vi "MPDSnC Engine.vi"(0 "Notifier Name":string, 11 "COM Port":string[](array[string])) -> ()   [LabVIEW 2025]
uses:
  AOTF Controls/AOTF Lines Lines Control.ctl
  AOTF Controls/AOTF Notifier Element.ctl
  AOTF Controls/AOTF Actions.ctl
  <vilib>/Utility/error.llb/Trim Whitespace One-Sided.vi
  <vilib>/Instr/_visa.llb/VISA Configure Serial Port (Instr).vi
panel:
  in  "Line On/Off":bool
  in  "Laser Wavelength (nm)":string
  out "Write Response":string
  in  "Blank":bool
  in  "Quit":bool
  in  "Power":dbl(slide) scale=0.0..100.0
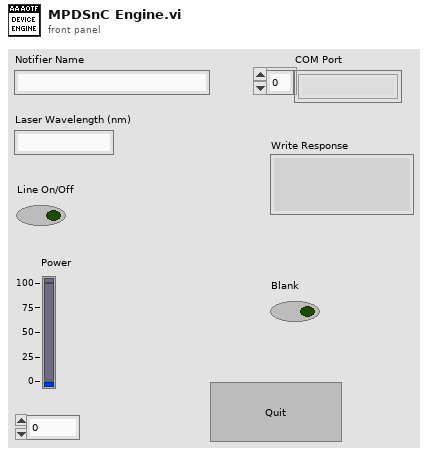
[diagram p1: front panel]
types:
  T1 = typedef "AOTF Notifier Element.ctl" = cluster{"AOTF Action":T2, "Laser Line":string, "Power (%)":dbl, "Beam Blank On/Off":bool, "Line On/Off":bool, "Error":errorcluster, "Wavelengths (nm)":string[]}
  T2 = typedef "AOTF Actions.ctl" = enum16{"Error Check", "Blank", "Line On/Off", "Set Power", "Status", "Quit"}
  T3 = typedef "AOTF Lines Lines Control.ctl" = cluster{"Wavelength":u16[], "AO Line":string[]}
  T4 = enum32{"Invalid", "Standard", "Closed", "Hidden", "Minimized", "Maximized"}
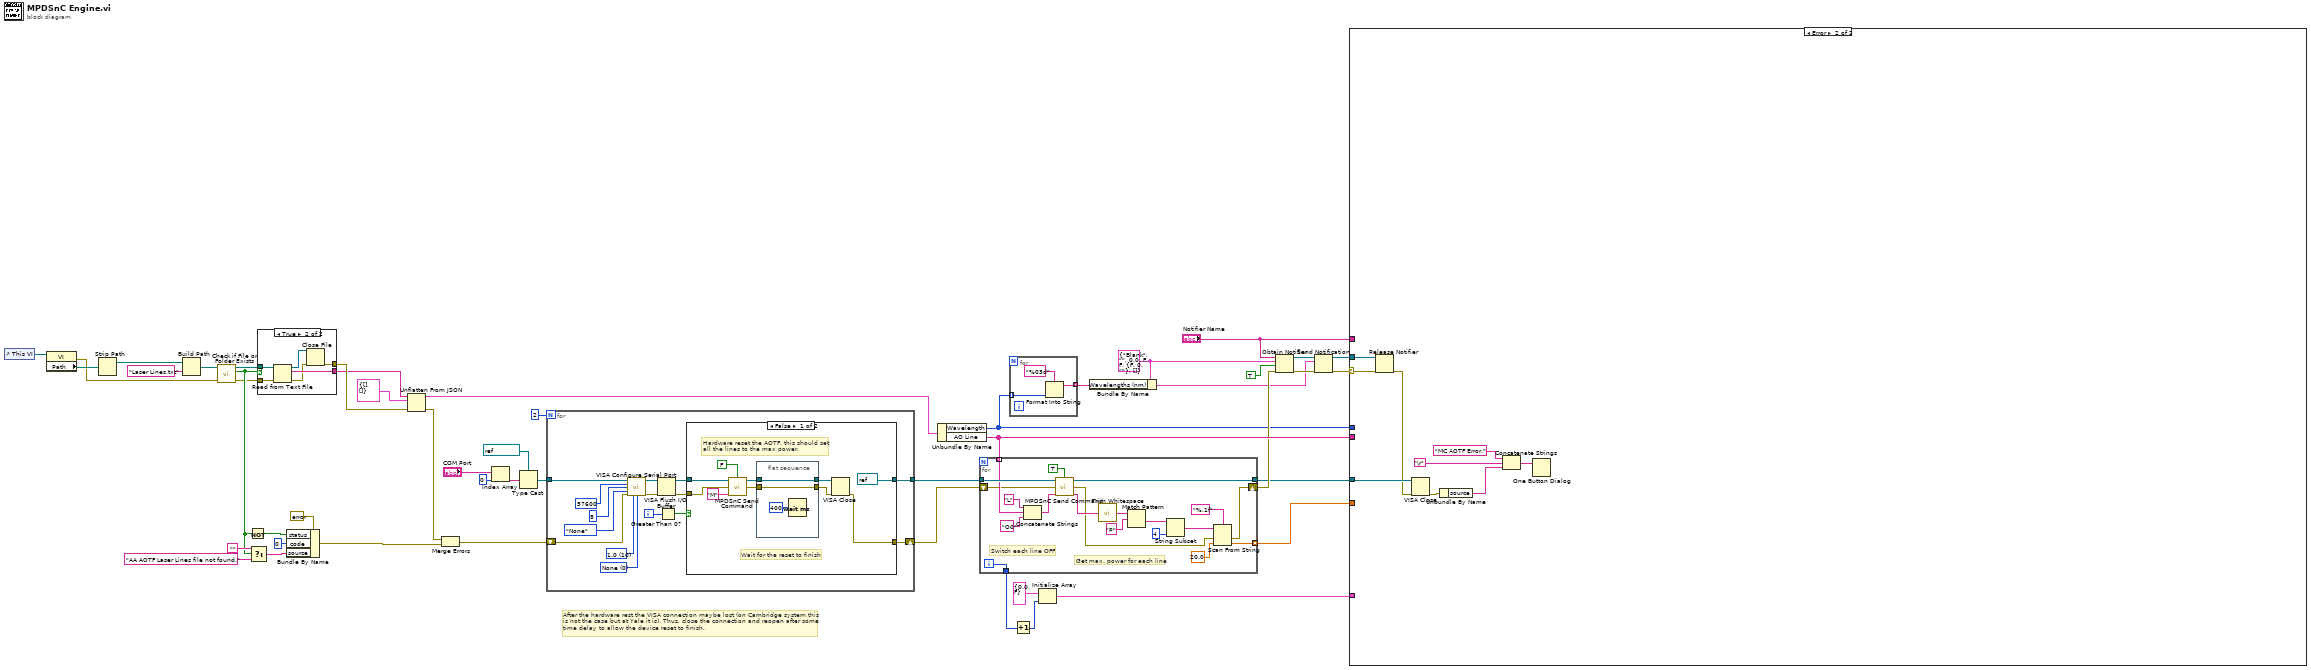
[diagram p0: block diagram]
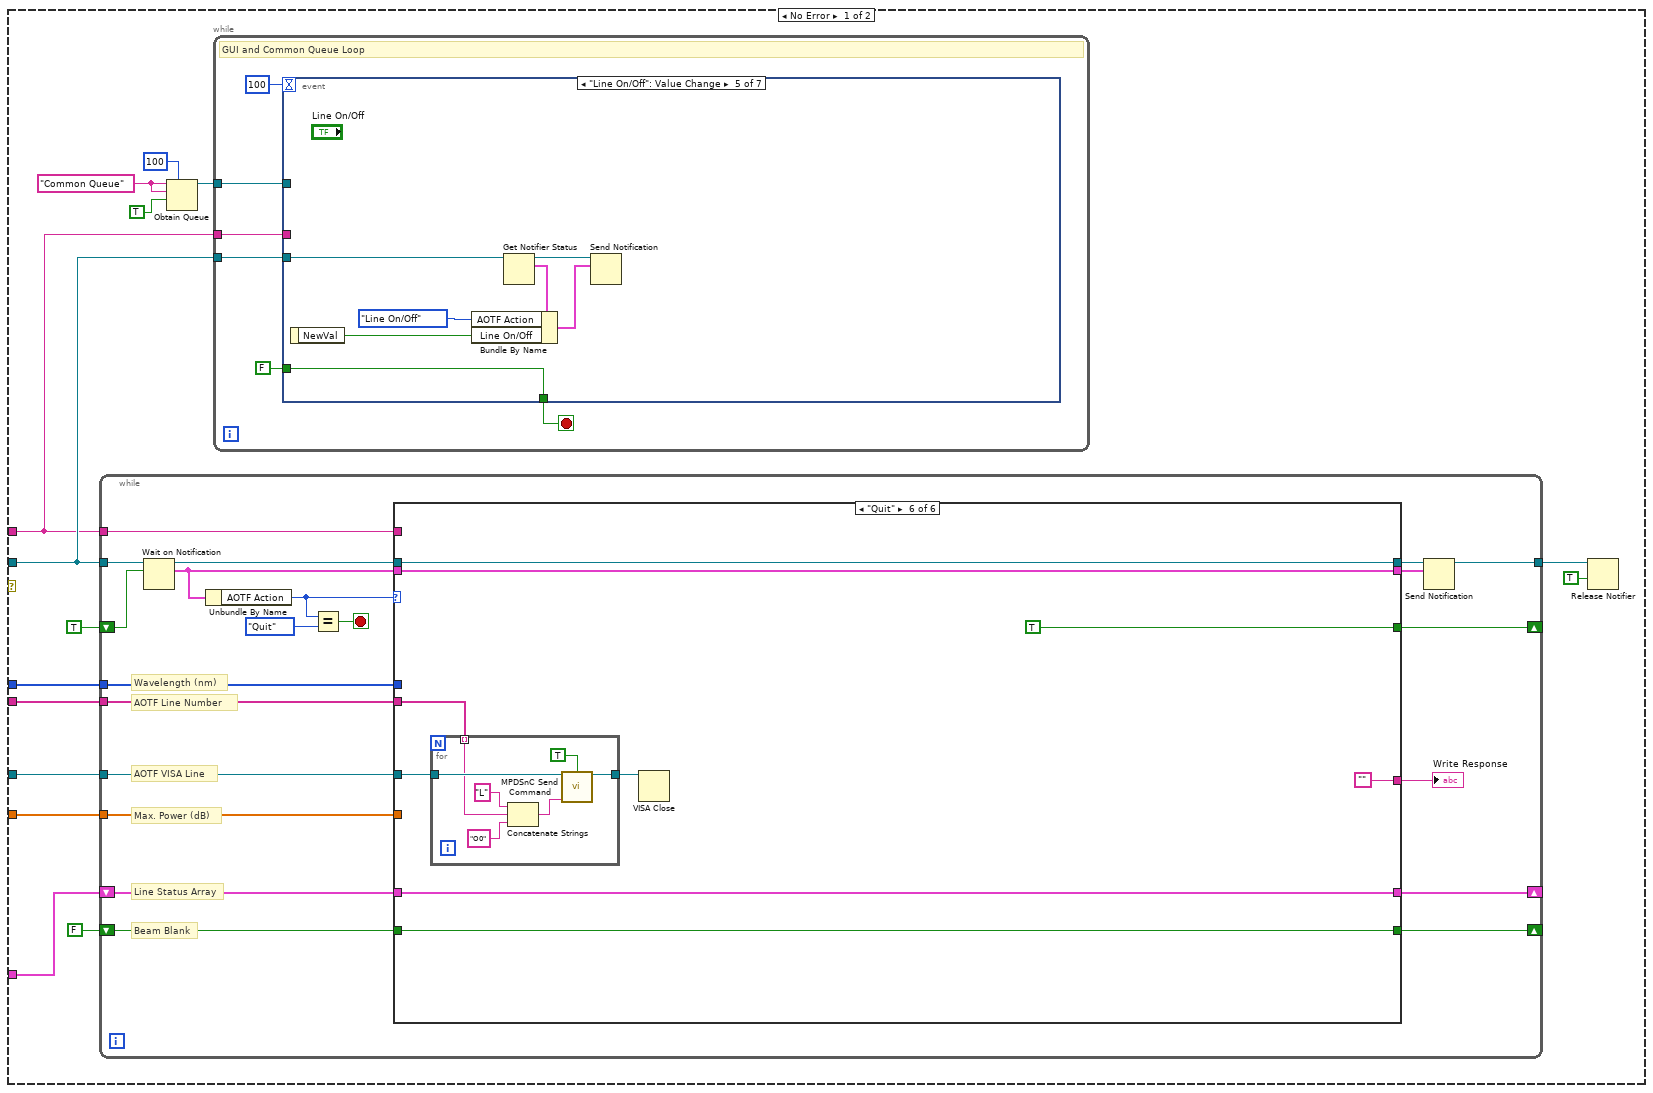
[diagram p3: hidden frame]
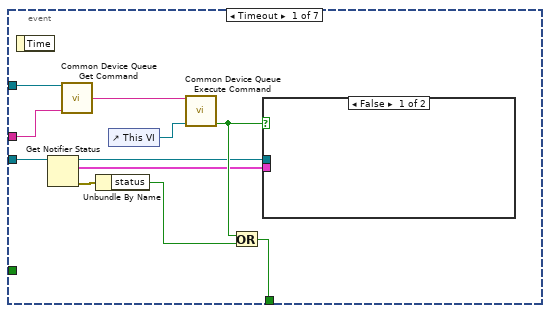
[diagram p4: hidden frame]
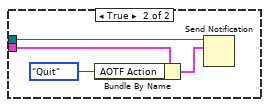
[diagram p5: hidden frame]
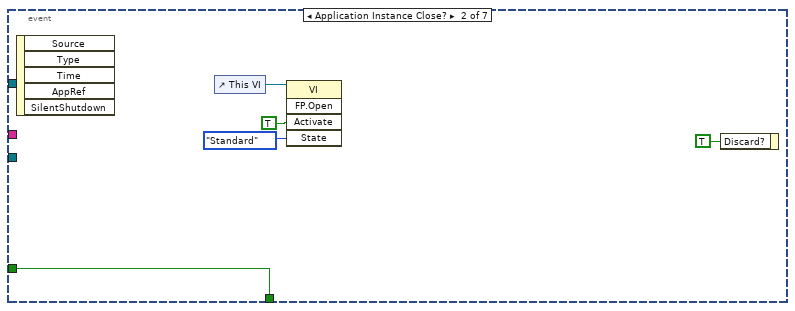
[diagram p6: hidden frame]
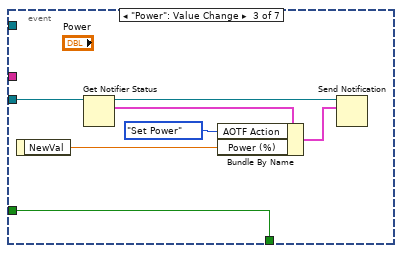
[diagram p7: hidden frame]
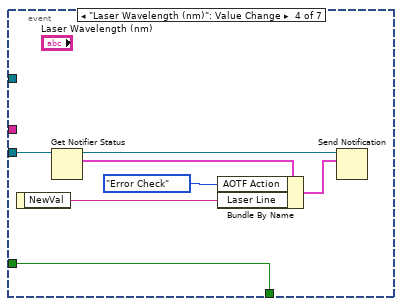
[diagram p8: hidden frame]
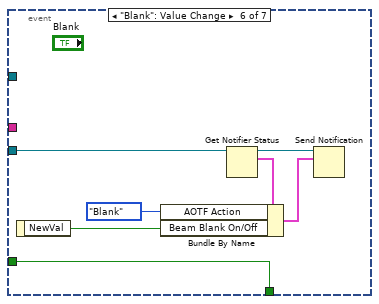
[diagram p9: hidden frame]
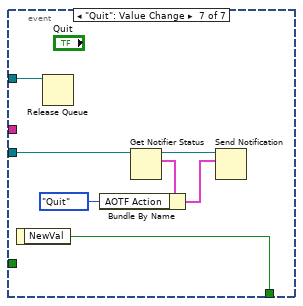
[diagram p10: hidden frame]
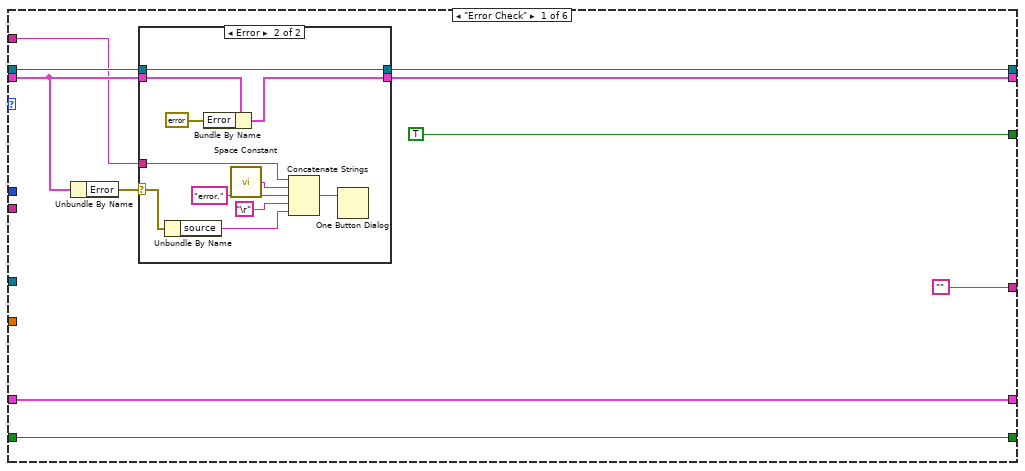
[diagram p11: hidden frame]
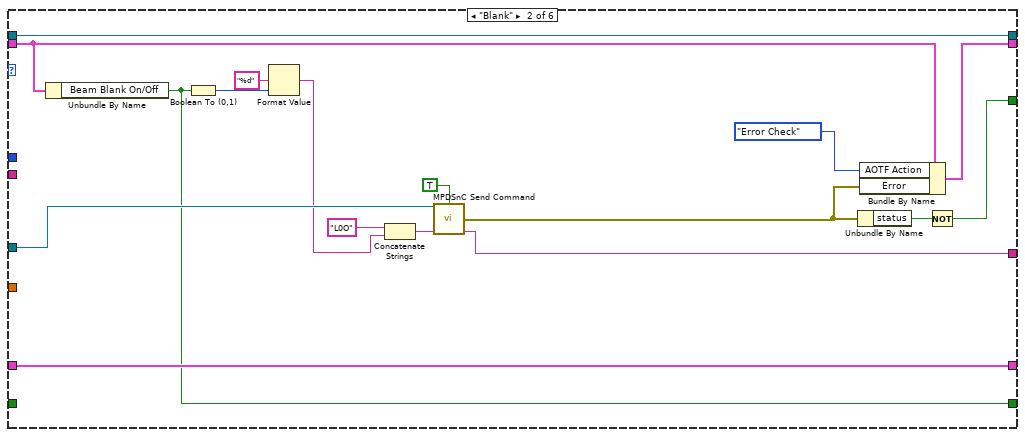
[diagram p13: hidden frame]
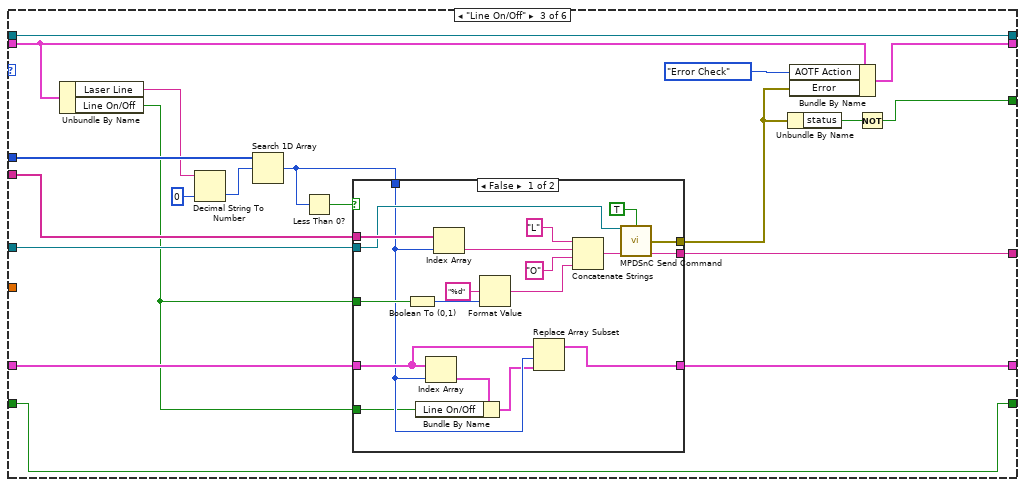
[diagram p14: hidden frame]
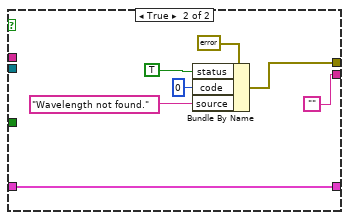
[diagram p15: hidden frame]
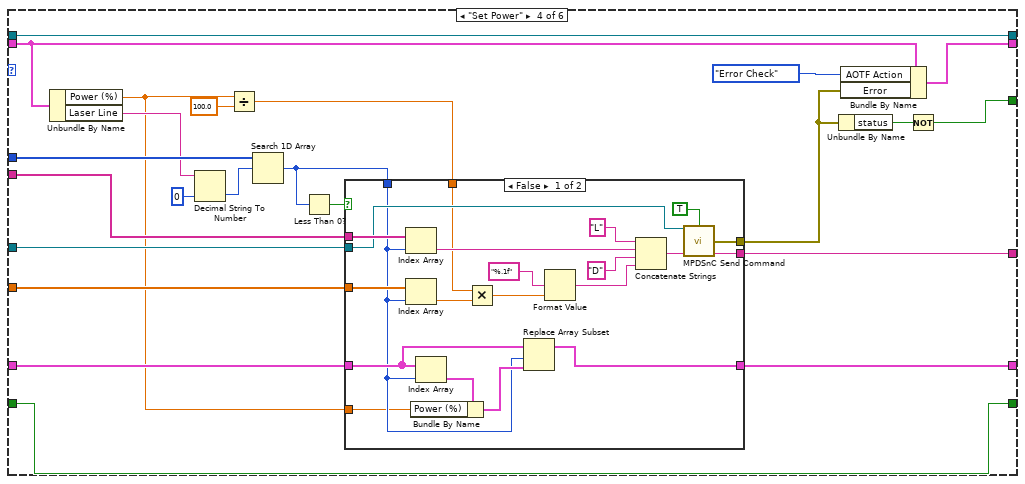
[diagram p16: hidden frame]
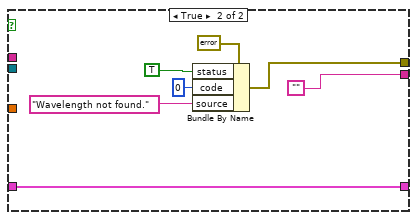
[diagram p17: hidden frame]
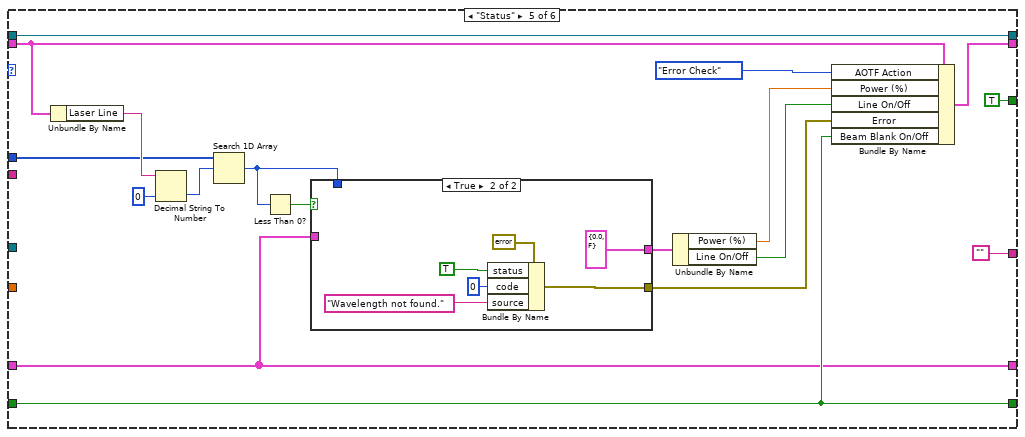
[diagram p18: hidden frame]
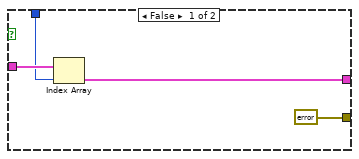
[diagram p19: hidden frame]
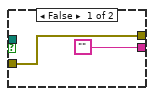
[diagram p20: hidden frame]
diagram:
  w3 = T1 {"AOTF Action"=enum."Blank", "Laser Line"="", "Power (%)"=0.0, "Beam Blank On/Off"=FALSE, "Line On/Off"=FALSE, "Error"={"status"=FALSE, "code"=0, "source"=""}, "Wavelengths (nm)"=[]} ("AOTFQueueCtrl")
  # "After the hardware rest the VISA connection maybe lost (on Cambridge system this\nis not the case but at Yale it is). Thus, close the connection and reopen after some\ntime delay to allow the device reset to finish."
  n1 = control-ref of="This VI"() -> (w48:refnum<vi>)
  n2 = property class="VI"(reference=w48) -> (error out=w35:errorcluster, "Path"=w47:path)  [unwired: 1 in, 1 out]
  n3 = Strip Path(path=w47) -> (stripped path=w46:path)  [unwired: 1 out]
  n4 = Build Path(base path=w46, name or relative path="Laser Lines.txt") -> (appended path=w44:path)
  n5 = call <vilib>:"Check if File or Folder Exists.vi"("error in (no error)"=w35, "path"=w44) -> ("error out"=w34:errorcluster, "file or folder exists?"=w37:bool, "dup path"=w36:path)  [unwired: 7 in]
  n6 = Not(x=w37) -> (.not. x?=w42:bool)
  n7 = Select(t="", s=w37, f="AA AOTF Laser Lines file not found." ("source")) -> (s? t:f=w38:string)
  n8 = case shown="True" w37 {
    tunnel: w36 -> [_ w56]
    tunnel: ["" w55] -> w30
    tunnel: w34 -> [w49 w53]
    tunnel: [w49 w51] -> w33
    frame False {
    }
    frame True {
      n9 = Read from Text File(file (use dialog)=w56, error in=w53) -> (refnum out=w54:refnum<file>, text=w55:string, error out=w52:errorcluster)  [unwired: 2 in, 1 out]
      n10 = Close File(refnum=w54, error in=w52) -> (error out=w51:errorcluster)  [unwired: 1 out]
    }
  }
  n11 = Bundle By Name(cluster=errorcluster {"status"=FALSE, "code"=0, "source"=""} ("Error"), "status"=w42, "code"=0, "source"=w38) -> (w31:errorcluster)
  n12 = Unflatten From JSON(JSON string=w30, type and defaults=T3 {"Wavelength"=[], "AO Line"=[]} ("Laser Lines"), error in (no error)=w33) -> (value=w28:T3, error out=w32:errorcluster)  [unwired: 4 in]
  n13 = Merge Errors(w32, w31) -> (w24:errorcluster)
  n14 = Index Array(array="COM Port", index=0) -> (element=w13:string)
  n15 = Type Cast(type=refnum<visa-resource-name> "COM6" ("reference"), x=w13) -> (*(type *) &x=w9:refnum<visa-resource-name>)
  n16 = for {
    N: 2 -> [_]
    tunnel: [w63] -> w26
    shift-right: [w61] -> w25
    shift-left: w24 -> [w60]
    tunnel: w9 -> [w57]
    i -> [w59]
    w71 = u16 0 items=["None", "XON/XOFF", "RTS/CTS", "XON/XOFF & RTS/CTS", "DTR/DSR", "XON/XOFF & DTR/DSR"] ("flow control (0:none)")
    w70 = u16 10 items=["1.0"=10, "1.5"=15, "2.0"=20] ("stop bits (10: 1 bit)")
    n17 = call-poly "VISA Configure Serial Port"("VISA resource name"=w57, "baud rate (9600)"=u32 57600, "data bits (8)"=u16 8, "parity (0:none)"=enum16{"None", "Odd", "Even", "Mark", "Space"}."None", "error in (no error)"=w60, "stop bits (10: 1 bit)"=w70, "flow control (0:none)"=w71) -> ("VISA resource name out"=w66:refnum<visa-resource-name>, "error out"=w65:errorcluster)  [unwired: 7 in]
    n18 = VISA Flush I/O Buffer(VISA resource name=w66, error in (no error)=w65) -> (VISA resource name out=w64:refnum<visa-resource-name>, error out=w62:errorcluster)  [unwired: 1 in]
    n19 = Greater Than 0?(x=w59) -> (x > 0?=w58:bool)
    n20 = case shown="False" w58 {
      tunnel: w64 -> [w81 w86]
      tunnel: [refnum<visa-resource-name> refnum ("VISA resource name") w86] -> w63
      tunnel: w62 -> [w80 w85]
      tunnel: [w73 w85] -> w61
      frame False {
        # "Wait for the reset to finish"
        # "Hardware reset the AOTF, this should set\nall the lines to the max power."
        n21 = call "MPDSnC Send Command.vi"("VISA Ref"=w81, "Wait for Reply?"=FALSE, "Error In"=w80, "Command"="M") -> ("VISA Ref Out"=w77:refnum<visa-resource-name>, "Error Out"=w76:errorcluster)  [unwired: 9 in, 1 out]
        n22 = flat-sequence {
          tunnel: [w84] -> w75
          tunnel: w77 -> [w84]
          tunnel: w76 -> [w82]
          tunnel: [w82] -> w74
          frame #0 {
            n23 = Wait (ms)(milliseconds to wait=u32 400) -> ()  [unwired: 1 out]
          }
        }
        n24 = VISA Close(VISA resource name=w75, error in (no error)=w74) -> (error out=w73:errorcluster)
      }
      frame True {
      }
    }
  }
  n25 = Unbundle By Name(w28) -> ("Wavelength"=w1:u16[], "AO Line"=w27:string[])
  n26 = for {
    tunnel: w26 -> [w105]
    tunnel: w27 -> [w103] mode=indexing
    tunnel: [w99] -> w19
    tunnel: [w92] -> w20 mode=indexing
    shift-right: [w88] -> w23
    shift-left: w25 -> [w90]
    tunnel: [w87] -> w17
    i -> [w87]
    # "Get max. power for each line"
    # "Switch each line OFF"
    n27 = Concatenate Strings("L", w103, "O0" ("string")) -> (w102:string)
    n28 = call "MPDSnC Send Command.vi"("VISA Ref"=w105, "Wait for Reply?"=TRUE, "Error In"=w90, "Command"=w102) -> ("VISA Ref Out"=w99:refnum<visa-resource-name>, "Error Out"=w89:errorcluster, "Response"=w100:string)  [unwired: 9 in]
    n29 = call <vilib>:"Trim Whitespace.vi"("string"=w100) -> ("trimmed string"=w98:string)  [unwired: 1 in]
    n30 = Match Pattern(string=w98, regular expression="P") -> (after substring=w96:string)  [unwired: 1 in, 3 out]
    n31 = String Subset(string=w96, length (rest)=4 ("length (rest)")) -> (substring=w94:string)  [unwired: 1 in]
    n32 = Scan From String(format string="%.1f", input string=w94, error in=w89, default 1=20.0 ("default value 1")) -> (error out=w88:errorcluster, output 1=w92:dbl)  [unwired: 1 in, 2 out]
  }
  n33 = for {
    tunnel: w1 -> [w109] mode=indexing
    tunnel: [w108] -> w8 mode=indexing
    n34 = Format Into String(format string="%03d", w109) -> (resulting string=w108:string)  [unwired: 2 in, 1 out]
  }
  n35 = Increment(x=w17) -> (x+1=w16:i32)
  n36 = Initialize Array(cluster{"Power (%)":dbl, "Line On/Off":bool} {"Power (%)"=0.0, "Line On/Off"=FALSE} ("Line Staus Cluster"), w16) -> (w15:cluster{"Power (%)":dbl, "Line On/Off":bool}[])
  n37 = Bundle By Name(cluster=w3, "Wavelengths (nm)"=w8) -> (w2:T1)
  n38 = Obtain Notifier(name (unnamed)="Notifier Name", notification data type=w3, create if not found? (T)=TRUE, error in (no error)=w23) -> (notifier out=w7:refnum<notifier>, error out=w6:errorcluster)  [unwired: 1 out]
  n39 = Send Notification(notification=w2, notifier=w7, error in (no error)=w6) -> (notifier out=w5:refnum<notifier>, error out=w4:errorcluster)
  n40 = case shown="Error" w4 {
    selector: w4 -> [_ w395]
    tunnel: w5 -> [w120 w396]
    tunnel: "Notifier Name" -> [w116 _]
    tunnel: w1 -> [w115 _]
    tunnel: w27 -> [w114 _]
    tunnel: w20 -> [w113 _]
    tunnel: w19 -> [w112 w390]
    tunnel: w15 -> [w111 _]
    frame No Error {
      w124 = "Common Queue" ("Unique Notifier Name")
      n41 = while {
        tunnel: w120 -> [w206]
        shift-right: [w197] -> _
        shift-left: TRUE ("ignore previous (F)") -> [w205]
        tunnel: [w196] -> w118
        tunnel: w116 -> [w195]
        tunnel: w115 -> [w194]
        tunnel: w114 -> [w193]
        tunnel: w113 -> [w192]
        tunnel: w112 -> [w191]
        shift-right: [w186] -> _
        shift-left: w111 -> [w189]
        shift-right: [w187] -> _
        shift-left: FALSE -> [w188]
        stop <- w200 stop-if-true
        # "Wavelength (nm)"
        # "AOTF Line Number"
        # "Line Status Array"
        # "Beam Blank"
        # "AOTF VISA Line"
        # "Max. Power (dB)"
        n42 = Wait on Notification(notifier=w206, ignore previous (F)=w205) -> (notifier out=w204:refnum<notifier>, notification=w203:T1)  [unwired: 2 in, 2 out]
        n43 = Unbundle By Name(w203) -> ("AOTF Action"=w202:T2)
        n44 = Equal?(x=w202, y=AOTF_Actions."Quit") -> (x = y?=w200:bool)
        n45 = case shown="\"Quit\"" w202 {
          tunnel: w204 -> [w216 w246 w262 w315 w360 w380]
          tunnel: w203 -> [w214 w245 w264 w311 w355 w379]
          tunnel: [w212 w246 w262 w315 w360 w380] -> w199
          tunnel: [w211 w244 w263 w310 w351 w379] -> w198
          tunnel: [TRUE w241 w251 w309 TRUE TRUE] -> w197
          tunnel: w195 -> [w213 _ _ _ _ _]
          tunnel: w194 -> [_ _ w259 w306 w356 _]
          tunnel: w193 -> [_ _ w256 w302 _ w374]
          tunnel: w192 -> [_ _ _ w299 _ _]
          tunnel: w191 -> [_ w239 w255 w298 _ w373]
          tunnel: ["" w232 w253 w297 "" ""] -> w190
          tunnel: w189 -> [w208 w231 w250 w296 w344 w376]
          tunnel: w188 -> [w207 _ w248 w293 w345 w375]
          tunnel: [w207 w230 w248 w293 w345 w375] -> w187
          tunnel: [w208 w231 w249 w294 w344 w376] -> w186
          frame "Error Check" {
            n46 = Unbundle By Name(w214) -> ("Error"=w215:errorcluster)
            n47 = case shown="Error" w215 {
              selector: w215 -> [_ w222]
              tunnel: w214 -> [w217 w226]
              tunnel: [w218 w224] -> w212
              tunnel: w216 -> [w218 w224]
              tunnel: w213 -> [_ w221]
              tunnel: [w217 w223] -> w211
              frame No Error {
              }
              frame Error {
                n48 = Unbundle By Name(w222) -> ("source"=w220:string)
                n49 = Bundle By Name(cluster=w226, "Error"=errorcluster {"status"=FALSE, "code"=0, "source"=""}) -> (w223:T1)
                n50 = call <vilib>:"Space Constant.vi"() -> ("String"=w229:string)
                n51 = Concatenate Strings(w221, w229, "error." ("string"), "\r", w220) -> (w227:string)
                n52 = One Button Dialog(message=w227) -> ()  [unwired: 1 in, 1 out]
              }
            }
          }
          frame "Blank" {
            n53 = Unbundle By Name(w245) -> ("Beam Blank On/Off"=w230:bool)
            n54 = Boolean To (0,1)(Boolean=w230) -> (0, 1=w235:i16)
            n55 = Format Value(format string="%d", value (0)=w235) -> (output string=w233:string)  [unwired: 1 in]
            n56 = Concatenate Strings("L0O", w233) -> (w236:string)
            n57 = call "MPDSnC Send Command.vi"("VISA Ref"=w239, "Wait for Reply?"=TRUE, "Command"=w236) -> ("Error Out"=w240:errorcluster, "Response"=w232:string)  [unwired: 10 in, 1 out]
            n58 = Unbundle By Name(w240) -> ("status"=w242:bool)
            n59 = Bundle By Name(cluster=w245, "AOTF Action"=AOTF_Actions."Error Check", "Error"=w240) -> (w244:T1)
            n60 = Not(x=w242) -> (.not. x?=w241:bool)
          }
          frame "Line On/Off" {
            n61 = Unbundle By Name(w264) -> ("Laser Line"=w258:string, "Line On/Off"=w247:bool)
            n62 = Decimal String To Number(string=w258, default (0L)=u16 0 ("default (0 I32)")) -> (number=w261:u16)  [unwired: 1 in, 1 out]
            n63 = Search 1D Array(1D array=w259, element=w261) -> (index of element=w254:i32)  [unwired: 1 in]
            n64 = Less Than 0?(x=w254) -> (x < 0?=w257:bool)
            n65 = case shown="False" w257 {
              tunnel: w256 -> [w285 _]
              tunnel: [w280 w288] -> w252
              tunnel: w254 -> [w270 _]
              tunnel: w255 -> [w278 _]
              tunnel: [w277 ""] -> w253
              tunnel: w247 -> [w274 _]
              tunnel: w250 -> [w272 w286]
              tunnel: [w271 w286] -> w249
              tunnel: w247 -> [w267 _]
              frame False {
                n66 = Boolean To (0,1)(Boolean=w274) -> (0, 1=w276:i16)
                n67 = Index Array(array=w272, index=w270) -> (element=w269:cluster{"Power (%)":dbl, "Line On/Off":bool})
                n68 = Bundle By Name(cluster=w269, "Line On/Off"=w267) -> (w268:cluster{"Power (%)":dbl, "Line On/Off":bool})
                n69 = Index Array(array=w285, index=w270) -> (element=w284:string)
                n70 = Format Value(format string="%d", value (0)=w276) -> (output string=w273:string)  [unwired: 1 in]
                n71 = Replace Array Subset(array=w272, new element=w268, index=w270) -> (w271:cluster{"Power (%)":dbl, "Line On/Off":bool}[])
                n72 = Concatenate Strings("L", w284, "O", w273) -> (w281:string)
                n73 = call "MPDSnC Send Command.vi"("VISA Ref"=w278, "Wait for Reply?"=TRUE, "Command"=w281) -> ("Error Out"=w280:errorcluster, "Response"=w277:string)  [unwired: 10 in, 1 out]
              }
              frame True {
                n74 = Bundle By Name(cluster=errorcluster {"status"=FALSE, "code"=0, "source"=""} ("error out"), "status"=TRUE, "code"=0, "source"="Wavelength not found.") -> (w288:errorcluster)
              }
            }
            n75 = Unbundle By Name(w252) -> ("status"=w265:bool)
            n76 = Bundle By Name(cluster=w264, "AOTF Action"=AOTF_Actions."Error Check", "Error"=w252) -> (w263:T1)
            n77 = Not(x=w265) -> (.not. x?=w251:bool)
          }
          frame "Set Power" {
            n78 = Unbundle By Name(w311) -> ("Power (%)"=w295:dbl, "Laser Line"=w305:string)
            n79 = Decimal String To Number(string=w305, default (0L)=u16 0 ("default (0 I32)")) -> (number=w307:u16)  [unwired: 1 in, 1 out]
            n80 = Divide(x=w295, y=100.0) -> (x/y=w301:dbl)
            n81 = Search 1D Array(1D array=w306, element=w307) -> (index of element=w303:i32)  [unwired: 1 in]
            n82 = Less Than 0?(x=w303) -> (x < 0?=w304:bool)
            n83 = case shown="False" w304 {
              tunnel: w302 -> [w336 _]
              tunnel: [w329 w339] -> w300
              tunnel: w303 -> [w319 _]
              tunnel: w301 -> [w318 _]
              tunnel: w299 -> [w333 _]
              tunnel: w298 -> [w324 _]
              tunnel: [w323 ""] -> w297
              tunnel: w296 -> [w320 w337]
              tunnel: w295 -> [w317 _]
              tunnel: [w316 w337] -> w294
              frame False {
                n84 = Index Array(array=w336, index=w319) -> (element=w335:string)
                n85 = Index Array(array=w333, index=w319) -> (element=w331:dbl)
                n86 = Index Array(array=w320, index=w319) -> (element=w322:cluster{"Power (%)":dbl, "Line On/Off":bool})
                n87 = Bundle By Name(cluster=w322, "Power (%)"=w317) -> (w321:cluster{"Power (%)":dbl, "Line On/Off":bool})
                n88 = Multiply(x=w318, y=w331) -> (x*y=w326:dbl)
                n89 = Replace Array Subset(array=w320, new element=w321, index=w319) -> (w316:cluster{"Power (%)":dbl, "Line On/Off":bool}[])
                n90 = Format Value(format string="%.1f", value (0)=w326) -> (output string=w325:string)  [unwired: 1 in]
                n91 = Concatenate Strings("L", w335, "D", w325) -> (w330:string)
                n92 = call "MPDSnC Send Command.vi"("VISA Ref"=w324, "Wait for Reply?"=TRUE, "Command"=w330) -> ("Error Out"=w329:errorcluster, "Response"=w323:string)  [unwired: 10 in, 1 out]
              }
              frame True {
                n93 = Bundle By Name(cluster=errorcluster {"status"=FALSE, "code"=0, "source"=""} ("error out"), "status"=TRUE, "code"=0, "source"="Wavelength not found.") -> (w339:errorcluster)
              }
            }
            n94 = Unbundle By Name(w300) -> ("status"=w312:bool)
            n95 = Bundle By Name(cluster=w311, "AOTF Action"=AOTF_Actions."Error Check", "Error"=w300) -> (w310:T1)
            n96 = Not(x=w312) -> (.not. x?=w309:bool)
          }
          frame "Status" {
            n97 = Unbundle By Name(w355) -> ("Laser Line"=w357:string)
            n98 = Decimal String To Number(string=w357, default (0L)=u16 0 ("default (0 I32)")) -> (number=w358:u16)  [unwired: 1 in, 1 out]
            n99 = Search 1D Array(1D array=w356, element=w358) -> (index of element=w353:i32)  [unwired: 1 in]
            n100 = Less Than 0?(x=w353) -> (x < 0?=w354:bool)
            n101 = case shown="True" w354 {
              tunnel: w344 -> [w365 _]
              tunnel: [errorcluster {"status"=FALSE, "code"=0, "source"=""} ("error out") w367] -> w349
              tunnel: w353 -> [w364 _]
              tunnel: [w363 cluster{"Power (%)":dbl, "Line On/Off":bool} {"Power (%)"=0.0, "Line On/Off"=FALSE} ("Line Staus Cluster")] -> w348
              frame False {
                n102 = Index Array(array=w365, index=w364) -> (element=w363:cluster{"Power (%)":dbl, "Line On/Off":bool})
              }
              frame True {
                n103 = Bundle By Name(cluster=errorcluster {"status"=FALSE, "code"=0, "source"=""} ("error out"), "status"=TRUE, "code"=0, "source"="Wavelength not found.") -> (w367:errorcluster)
              }
            }
            n104 = Unbundle By Name(w348) -> ("Power (%)"=w347:dbl, "Line On/Off"=w346:bool)
            n105 = Bundle By Name(cluster=w355, "AOTF Action"=AOTF_Actions."Error Check", "Power (%)"=w347, "Line On/Off"=w346, "Error"=w349, "Beam Blank On/Off"=w345) -> (w351:T1)
          }
          frame "Quit" {
            n106 = for {
              tunnel: w373 -> [w386]
              tunnel: w374 -> [w384] mode=indexing
              tunnel: [w381] -> w372
              n107 = Concatenate Strings("L", w384, "O0" ("string")) -> (w383:string)
              n108 = call "MPDSnC Send Command.vi"("VISA Ref"=w386, "Wait for Reply?"=TRUE, "Command"=w383) -> ("VISA Ref Out"=w381:refnum<visa-resource-name>)  [unwired: 10 in, 2 out]
            }
            n109 = VISA Close(VISA resource name=w372) -> ()  [unwired: 1 in, 1 out]
          }
        }
        "Write Response" <- w190
        n110 = Send Notification(notification=w198, notifier=w199) -> (notifier out=w196:refnum<notifier>)  [unwired: 1 in, 1 out]
      }
      n111 = Obtain Queue(max queue size (-1, unlimited)=100, name (unnamed)=w124, element data type=w124, create if not found? (T)=TRUE) -> (queue out=w121:refnum<queue>)  [unwired: 1 in, 2 out]
      n112 = while {
        tunnel: w121 -> [w129]
        tunnel: w116 -> [w127]
        tunnel: w120 -> [w128]
        stop <- w126 stop-if-true
        # "GUI and Common Queue Loop"
        n113 = event shown="[4] \"Line On/Off\": Value Change" {
          selector: _ -> [_ _ _ _ _ _ _]
          dyn-events: _ -> [_ _ _ _ _ _ _]
          timeout: 100 -> [_ _ _ _ _ _ _]
          tunnel: w129 -> [w136 _ _ _ _ _ w185]
          tunnel: w128 -> [w132 _ w153 w160 w167 w177 w184]
          tunnel: w127 -> [w135 _ _ _ _ _ _]
          tunnel: [w134 w150 w157 w164 w171 w178 w182] -> w126
          tunnel: FALSE -> [_ w150 w157 w164 w171 w178 _]
          event Timeout {
            n114 = event-data() -> ()  [unwired: 1 in, 1 out]
            n115 = Get Notifier Status(notifier=w132) -> (notifier out=w131:refnum<notifier>, current notification=w133:T1, error out=w141:errorcluster)  [unwired: 1 in, 2 out]
            n116 = call "Common Device Queue Get Command.vi"("Common Queue"=w136, "Notifier Name"=w135) -> ("Command"=w140:string)  [unwired: 12 in, 1 out]
            n117 = Unbundle By Name(w141) -> ("status"=w138:bool)
            n118 = control-ref of="This VI"() -> (w139:refnum<vi>)
            n119 = call "Common Device Queue Execute Command.vi"("Common Command"=w140, "VI Refnum"=w139) -> ("Quit?"=w137:bool)  [unwired: 12 in, 1 out]
            n120 = Or(x=w137, y=w138) -> (x .or. y?=w134:bool)
            n121 = case shown="False" w137 {
              tunnel: w131 -> [_ w145]
              tunnel: w133 -> [_ w144]
              frame False {
              }
              frame True {
                n122 = Bundle By Name(cluster=w144, "AOTF Action"=AOTF_Actions."Quit") -> (w143:T1)
                n123 = Send Notification(notification=w143, notifier=w145) -> ()  [unwired: 1 in, 2 out]
              }
            }
          }
          event Application Instance Close? {
            n124 = event-data() -> ()  [unwired: 1 in, 5 out]
            n125 = control-ref of="This VI"() -> (w147:refnum<vi>)
            n126 = invoke class="VI" method="FP.Open"(reference=w147, "Activate"=TRUE ("Activate?"), "State"=T4."Standard") -> ()  [unwired: 2 in, 5 out]
            n127 = event-data("Discard?"=TRUE) -> ()  [unwired: 1 in, 1 out]
          }
          event "Power": Value Change {
            n128 = event-data() -> ("NewVal"=w155:dbl)  [unwired: 1 in]
            n129 = Get Notifier Status(notifier=w153) -> (notifier out=w151:refnum<notifier>, current notification=w152:T1)  [unwired: 1 in, 3 out]
            n130 = Bundle By Name(cluster=w152, "AOTF Action"=AOTF_Actions."Set Power", "Power (%)"=w155) -> (w154:T1)
            n131 = Send Notification(notification=w154, notifier=w151) -> ()  [unwired: 1 in, 2 out]
          }
          event "Laser Wavelength (nm)": Value Change {
            n132 = event-data() -> ("NewVal"=w162:string)  [unwired: 1 in]
            n133 = Get Notifier Status(notifier=w160) -> (notifier out=w158:refnum<notifier>, current notification=w159:T1)  [unwired: 1 in, 3 out]
            n134 = Bundle By Name(cluster=w159, "AOTF Action"=AOTF_Actions."Error Check", "Laser Line"=w162) -> (w161:T1)
            n135 = Send Notification(notification=w161, notifier=w158) -> ()  [unwired: 1 in, 2 out]
          }
          event "Line On/Off": Value Change {
            n136 = event-data() -> ("NewVal"=w166:bool)  [unwired: 1 in]
            n137 = Get Notifier Status(notifier=w167) -> (notifier out=w170:refnum<notifier>, current notification=w169:T1)  [unwired: 1 in, 3 out]
            n138 = Bundle By Name(cluster=w169, "AOTF Action"=AOTF_Actions."Line On/Off", "Line On/Off"=w166) -> (w165:T1)
            n139 = Send Notification(notification=w165, notifier=w170) -> ()  [unwired: 1 in, 2 out]
          }
          event "Blank": Value Change {
            n140 = event-data() -> ("NewVal"=w173:bool)  [unwired: 1 in]
            n141 = Get Notifier Status(notifier=w177) -> (notifier out=w176:refnum<notifier>, current notification=w175:T1)  [unwired: 1 in, 3 out]
            n142 = Bundle By Name(cluster=w175, "AOTF Action"=AOTF_Actions."Blank", "Beam Blank On/Off"=w173) -> (w172:T1)
            n143 = Send Notification(notification=w172, notifier=w176) -> ()  [unwired: 1 in, 2 out]
          }
          event "Quit": Value Change {
            n144 = event-data() -> ("NewVal"=w182:bool)  [unwired: 1 in]
            n145 = Release Queue(queue=w185) -> ()  [unwired: 2 in, 3 out]
            n146 = Get Notifier Status(notifier=w184) -> (notifier out=w183:refnum<notifier>, current notification=w181:T1)  [unwired: 1 in, 3 out]
            n147 = Bundle By Name(cluster=w181, "AOTF Action"=AOTF_Actions."Quit") -> (w179:T1)
            n148 = Send Notification(notification=w179, notifier=w183) -> ()  [unwired: 1 in, 2 out]
          }
        }
      }
      n149 = Release Notifier(notifier=w118, force destroy? (F)=TRUE) -> ()  [unwired: 1 in, 3 out]
    }
    frame Error {
      n150 = Release Notifier(notifier=w396, error in (no error)=w395) -> (error out=w389:errorcluster)  [unwired: 1 in, 2 out]
      n151 = VISA Close(VISA resource name=w390, error in (no error)=w389) -> (error out=w388:errorcluster)
      n152 = Unbundle By Name(w388) -> ("source"=w392:string)
      n153 = Concatenate Strings("MC AOTF Error.", "\r", w392) -> (w391:string)
      n154 = One Button Dialog(message=w391) -> ()  [unwired: 1 in, 1 out]
    }
  }
